vi "OPCUA AreAllTagsInitializedl.vi"(8 "error in (no error)":errorcluster, 11 "reference":refnum<k24>) -> (0 "error out":errorcluster, 1 "Initialized":bool, 3 "reference out":refnum<k24>)   [LabVIEW 2019]
uses:
  F:/src/HUTCDLSVN/Machine/CDL0100/TagEngine/LVOPCUA.NET/LVOPC.NETInterface/bin/Release/LVOPC.NETInterface.dll
  LVOPCUA.NET/LVOPC.NETInterface/bin/Release/LVOPC.NETInterface.dll
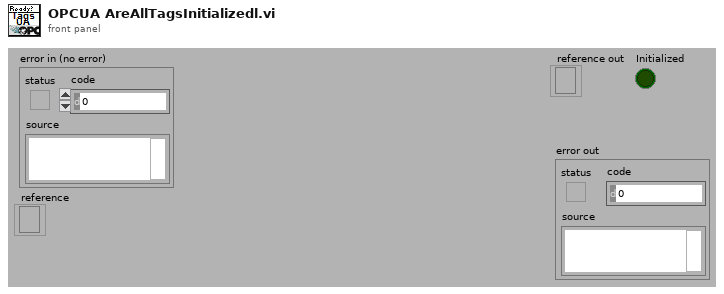
[diagram p1: front panel]
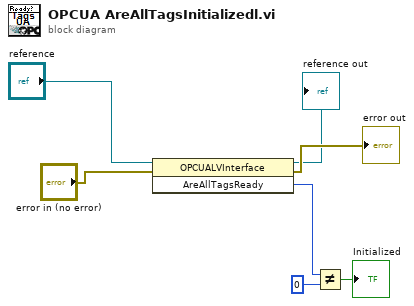
[diagram p0: block diagram]
diagram:
  n1 = invoke class="OPCUALVInterface" method="AreAllTagsReady"(reference="reference", error in="error in (no error)") -> (reference out=→"reference out":refnum<k24>, error out=→"error out":errorcluster, "AreAllTagsReady"=w4:i32)  [unwired: 1 in]
  n2 = Not Equal?(x=w4, y=0) -> (x != y?=→"Initialized":bool)
